vi "Query Output Status.vi"(6 "Settle (1mS)":u32=1, 8 "error in (no error)":errorcluster, 11 "VISA resource name":refnum<visa-resource-name>) -> (0 "error out":errorcluster, 2 "Output On":bool, 3 "VISA resource name out":refnum<visa-resource-name>)   [LabVIEW 2018, in "TDK-Lambda Z.lvlib"]
doc: "Queries output status of the power supply.\n True if the power supply output is On.\n False if the power supply output is Off."
uses:
  TDK-Lambda Z.lvlib
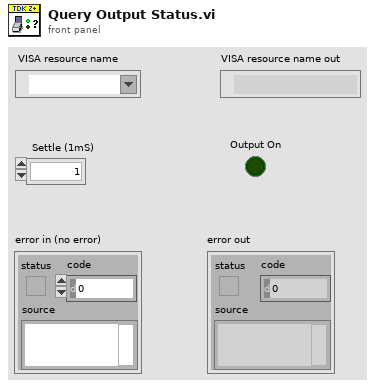
[diagram p1: front panel]
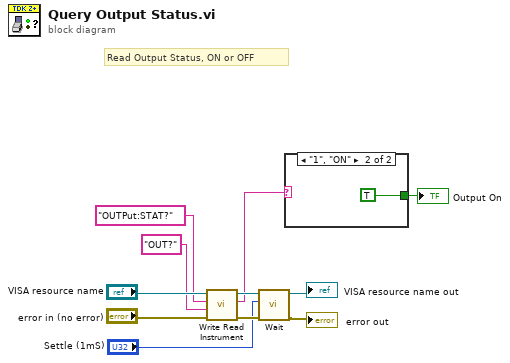
[diagram p0: block diagram]
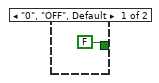
[diagram p2: hidden frame]
diagram:
  # "Read Output Status, ON or OFF"
  n1 = call "Write Read Instrument.vi"("error in (no error)"="error in (no error)", "GEN  Write Command/Query"="OUT?" ("format string"), "SCPI  Write Command/Query"="OUTPut:STAT?" ("format string"), "VISA resource name"="VISA resource name") -> ("error out"=w8:errorcluster, "Response"=w2:string, "VISA resource name out"=w9:refnum<visa-resource-name>)  [unwired: 5 in]
  n2 = call "Wait.vi"("error in (no error)"=w8, "Wait (1mS)"="Settle (1mS)", "VISA resource name"=w9) -> ("error out"=→"error out":errorcluster, "VISA resource name out"=→"VISA resource name out":refnum<visa-resource-name>)  [unwired: 7 in]
  n3 = case shown="\"1\", \"ON\"" w2 {
    tunnel: [FALSE TRUE] -> w1
    frame "0", "OFF", Default {
    }
    frame "1", "ON" {
    }
  }
  "Output On" <- w1
